vi "Create frame string.vi"(3 "Frame":T1 {"Data" format="%.0x"}) -> (1 "String":string)   [LabVIEW 2021, in "uCanDriver.lvlib" / "uCAN.lvclass"]
uses:
  uCAN.lvclass
  typedefs/frame.ctl
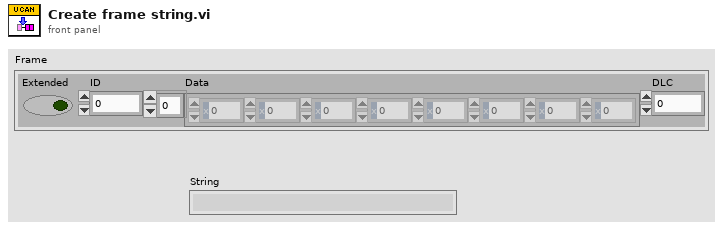
[diagram p1: front panel]
types:
  T1 = typedef "uCanDriver.lvlib/uCAN.lvclass/frame.ctl" = cluster{"Extended":bool, "ID":u32, "Data":u8[], "DLC":u8}
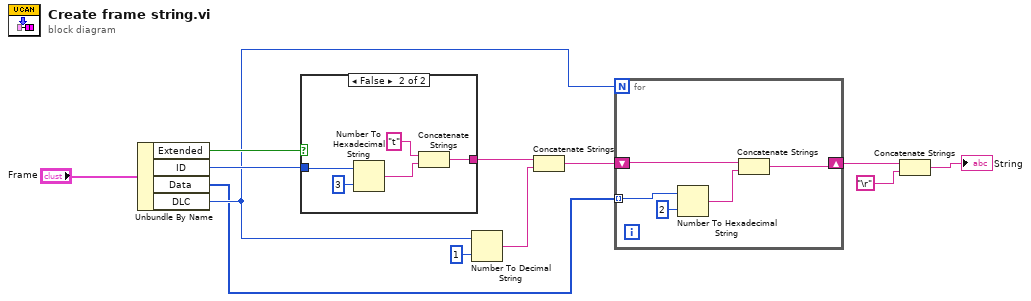
[diagram p0: block diagram]
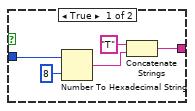
[diagram p2: hidden frame]
diagram:
  n1 = Unbundle By Name("Frame") -> ("Extended"=w11:bool, "ID"=w10:u32, "Data"=w4:u8[], "DLC"=w5:u8)
  n2 = case shown="False" w11 {
    tunnel: w10 -> [w17 w22]
    tunnel: [w13 w18] -> w8
    frame True {
      n3 = Number To Hexadecimal String(1:i16 8 ("width (-)"), 2:w17) -> (0:w14:string)
      n4 = Concatenate Strings("T" ("string"), w14) -> (w13:string)
    }
    frame False {
      n5 = Number To Hexadecimal String(1:i16 3 ("width (-)"), 2:w22) -> (0:w19:string)
      n6 = Concatenate Strings("t" ("string"), w19) -> (w18:string)
    }
  }
  n7 = Number To Decimal String(number=w5, width (-)=i16 1) -> (decimal integer string=w7:string)
  n8 = Concatenate Strings(w8, w7) -> (w6:string)
  n9 = for {
    N: w5 -> [_]
    tunnel: w4 -> [w24] mode=indexing
    shift-right: [w26] -> w3
    shift-left: w6 -> [w27]
    n10 = Number To Hexadecimal String(1:i16 2 ("width (-)"), 2:w24) -> (0:w23:string)
    n11 = Concatenate Strings(w27, w23) -> (w26:string)
  }
  n12 = Concatenate Strings(w3, "\r") -> (→"String":string)
